vi "Dashboard Main.vi"() -> ()   [LabVIEW 2012]
uses:
  <vilib>/event_ctls.llb/eventvkey.ctl
  <vilib>/Utility/config.llb/Read Key (String).vi
  <vilib>/Utility/config.llb/Read Key (I32).vi
  <vilib>/Utility/config.llb/Write Key (String).vi
  <vilib>/Utility/config.llb/Write Key (I32).vi
  <vilib>/Utility/config.llb/NI_LVConfig.lvlib
panel:
  out "Battery Value":dbl(slide) scale=0.0..14.0 scale format="%#_2e"
  out "Battery":sgl(graph)
  in  "Camera Settings":T1={"Frate Rate"=30, "Compression"=30, "Size"=1} {"Frate Rate" scale=1.0..30.0; "Size" items=["640x480", "320x240", "160x120"]}
  out "Mode":T2(ring)=enum."Auto Disabled"
  out "Camera IP":string
  out "JS1 Z":dbl(slide) scale=-1.0..1.0 scale format="%#_2e"
  out "JS2 Z":dbl(slide) scale=-1.0..1.0 scale format="%#_2e"
  out "Joystick 1":cluster{"X":dbl, "Y":dbl}[](graph)
  out "Joystick 2":cluster{"X":dbl, "Y":dbl}[](graph)
  out "JS Buttons 1":T3
  out "JS Buttons 2":T3
  out "MotorSlide4":dbl(slide) scale=-1.0..1.0 scale format="%#_2e"
  out "MotorSlide3":dbl(slide) scale=-1.0..1.0 scale format="%#_2e"
  out "MotorSlide2":dbl(slide) scale=-1.0..1.0 scale format="%#_2e"
  in  "MotorName3":string="Front Left"
  in  "MotorName4":string="Front Right"
  in  "MotorName1":string="Rear Left"
  in  "MotorName2":string="Rear Right"
  out "MotorChart4":dbl(graph)
  out "MotorChart3":dbl(graph)
  out "MotorChart2":dbl(graph)
  out "MotorSlide1":dbl(slide) scale=-1.0..1.0 scale format="%#_2e"
  out "MotorChart1":dbl(graph)
  out "Robot IP":string
  in  "Dashboard Tab":enum32{"Operation", "Test", "Checklist"}(tab)
  in  "Checkbox 2":bool
  in  "Checkbox 1":bool
  in  "Slider 1":dbl(slide) scale=0.0..100.0
  in  "Slider":dbl(slide) scale=0.0..100.0 scale format="%#_3g"
  in  "On/Off":bool caption="Solenoid"
  in  "Test Name":u16(ring) items=["Select the test to run...", "Example Test", "-------------------------------", "List of tests is built in robot code.", "Replace with your own automated tests."]
  in  "Test Tree":string(tree)
  in  "Motor":cluster{"Value":dbl, "Enable":bool} {"Value" scale=-1.0..1.0 scale format="%#_3g"}
  out "Progress":T4 {"Test Progress" scale=0.0..100.0}
  in  "Rev/Fwd":cluster{"Forward":bool, "Reverse":bool}
  in  "Ring":u16(ring) items=["Auto", "Fixed indoor", "Fixed outdoor 1", "Fixed outdoor 2", "Fixed fluorescent 1", "Fixed fluorescent 2", "Hold current"]
  in  "Listbox":i32(listbox)
  in  "Viewer":T5(tab)
  out "Mbps":dbl format="%#.1g"
  in  "Enable":bool
  in  "DB Camera Config":bool
  out "Mbps":bool
  out "fps":dbl format="%#.1g"
  out "Image Error Message":string="Timeout in Camera Communications"
  out "Camera Image":T6(plugin-control)
  out "Buttons 1":cluster{"1":bool, "2":bool, "3":bool}
  out "Kinect 1":cluster{"X":dbl, "Y":dbl, "Z":dbl} {"X" scale=1.0..-1.0; "Y" scale=1.0..-1.0; "Z" scale=1.0..-1.0}
  out "Buttons 2":cluster{"1":bool, "2":bool, "3":bool}
  out "Kinect 2":cluster{"X":dbl, "Y":dbl, "Z":dbl} {"X" scale=1.0..-1.0; "Y" scale=1.0..-1.0; "Z" scale=1.0..-1.0}
  out "Version":string
  out "Skeleton Picture":picture
  out "Players":i8
  out "Tree":string(tree)
  # "Drive & Motors"
  # "Robot IP:"
  # "Customize by placing controls and indicators here and name to match\nDashboard Variables on robot."
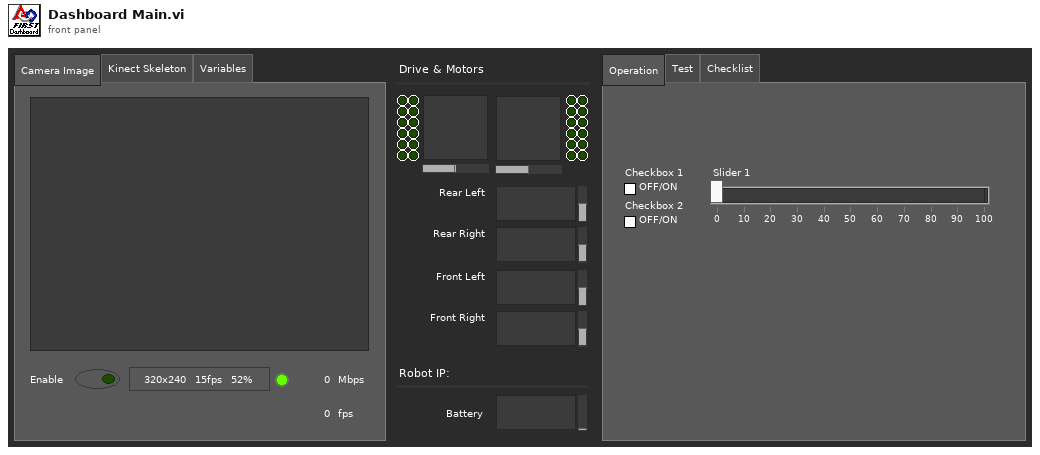
[diagram p1: front panel]
types:
  T1 = cluster{"Frate Rate":i32, "Compression":i32, "Size":u16}
  T2 = enum8{"Tele-Op Disabled", "Tele-Op Enabled", "Auto Disabled", "Auto Enabled", "Test Disabled", "Test Enabled", ""}
  T3 = cluster{bool, bool, bool, bool, bool, bool, bool, bool, bool, bool, bool, bool}
  T4 = cluster{"Test Progress":u8, "Test Progress Text":string}
  T5 = enum32{"Camera Image", "Kinect Skeleton", "Variables"}
  T6 = typedef "IMAQ Image.ctl" = refnum<image>
  T7 = typedef "Image Type" = u32
  T8 = typedef "LVBoundsTypeDef.ctl" = cluster{"Width":u32, "Height":u32}
  T9 = typedef "SkeletonTrackState.ctl" = enum32{"NotTracked", "PositionOnly", "Tracked"}
  T10 = cluster{"TrackingState":u8[], "Position":cluster{"x":sgl, "y":sgl, "z":sgl}, cluster{"x":sgl, "y":sgl, "z":sgl, sgl}[], "TrackState":T9}
  T11 = cluster{cluster{"ScaledToPercentRange":dbl, "ScaledToPercentRange":dbl, "ScaledToPercentRange":dbl}, cluster{bool, bool, bool}}[]
  T12 = cluster{cluster{"ScaledToPercentRange":dbl, "ScaledToPercentRange":dbl, "ScaledToPercentRange":dbl}, cluster{bool, bool, bool}}
  T13 = cluster{"ScaledToPercentRange":dbl, "ScaledToPercentRange":dbl, "ScaledToPercentRange":dbl}
  T14 = typedef "LVRectTypeDef.ctl" = cluster{"Left":i16, "Top":i16, "Right":i16, "Bottom":i16}
  T15 = cluster{"Competition mode":bool, "Robot Link":bool, "Autonomous":bool, "Enabled":bool, "E-Stop":bool, "Simulated":bool, "TestMode":bool, "Docked Window":bool}
  T16 = cluster{"Boolean Array[0]":bool, "Boolean Array[1]":bool, "Boolean Array[2]":bool, "Boolean Array[3]":bool, "Boolean Array[4]":bool, "Boolean Array[5]":bool, "Boolean Array[6]":bool, "Boolean Array[7]":bool, "Boolean Array[8]":bool, "Boolean Array[9]":bool, "Boolean Array[10]":bool, "Boolean Array[11]":bool}
  T17 = typedef "NI_LVConfig.lvlib/Config Data RefNum.ctl" = refnum<k1>
  T18 = typedef "eventvkey.ctl" = enum16{"ASCII", "Enter", "Return", "Shift", "Ctrl", "Alt", "Cmd", "Opt", "Caps", "NumLock", "Clear", "Break", "Up", "Down", "Left", "Right", "Insert", "Delete", "Home", "End", "PageUp", "PageDown", "Escape", "Help", "Pause", "ScrollLock", "F1", "F2", "F3", "F4", "F5", "F6", "F7", "F8", "F9", "F10", "F11", "F12", "F13", "F14", "F15", "F16", "F17", "F18", "F19", "F20", "F21", "F22", "F23", "F24", "Play", "VolumeUp", "VolumeDown", "Mute", "Two Byte Char"}
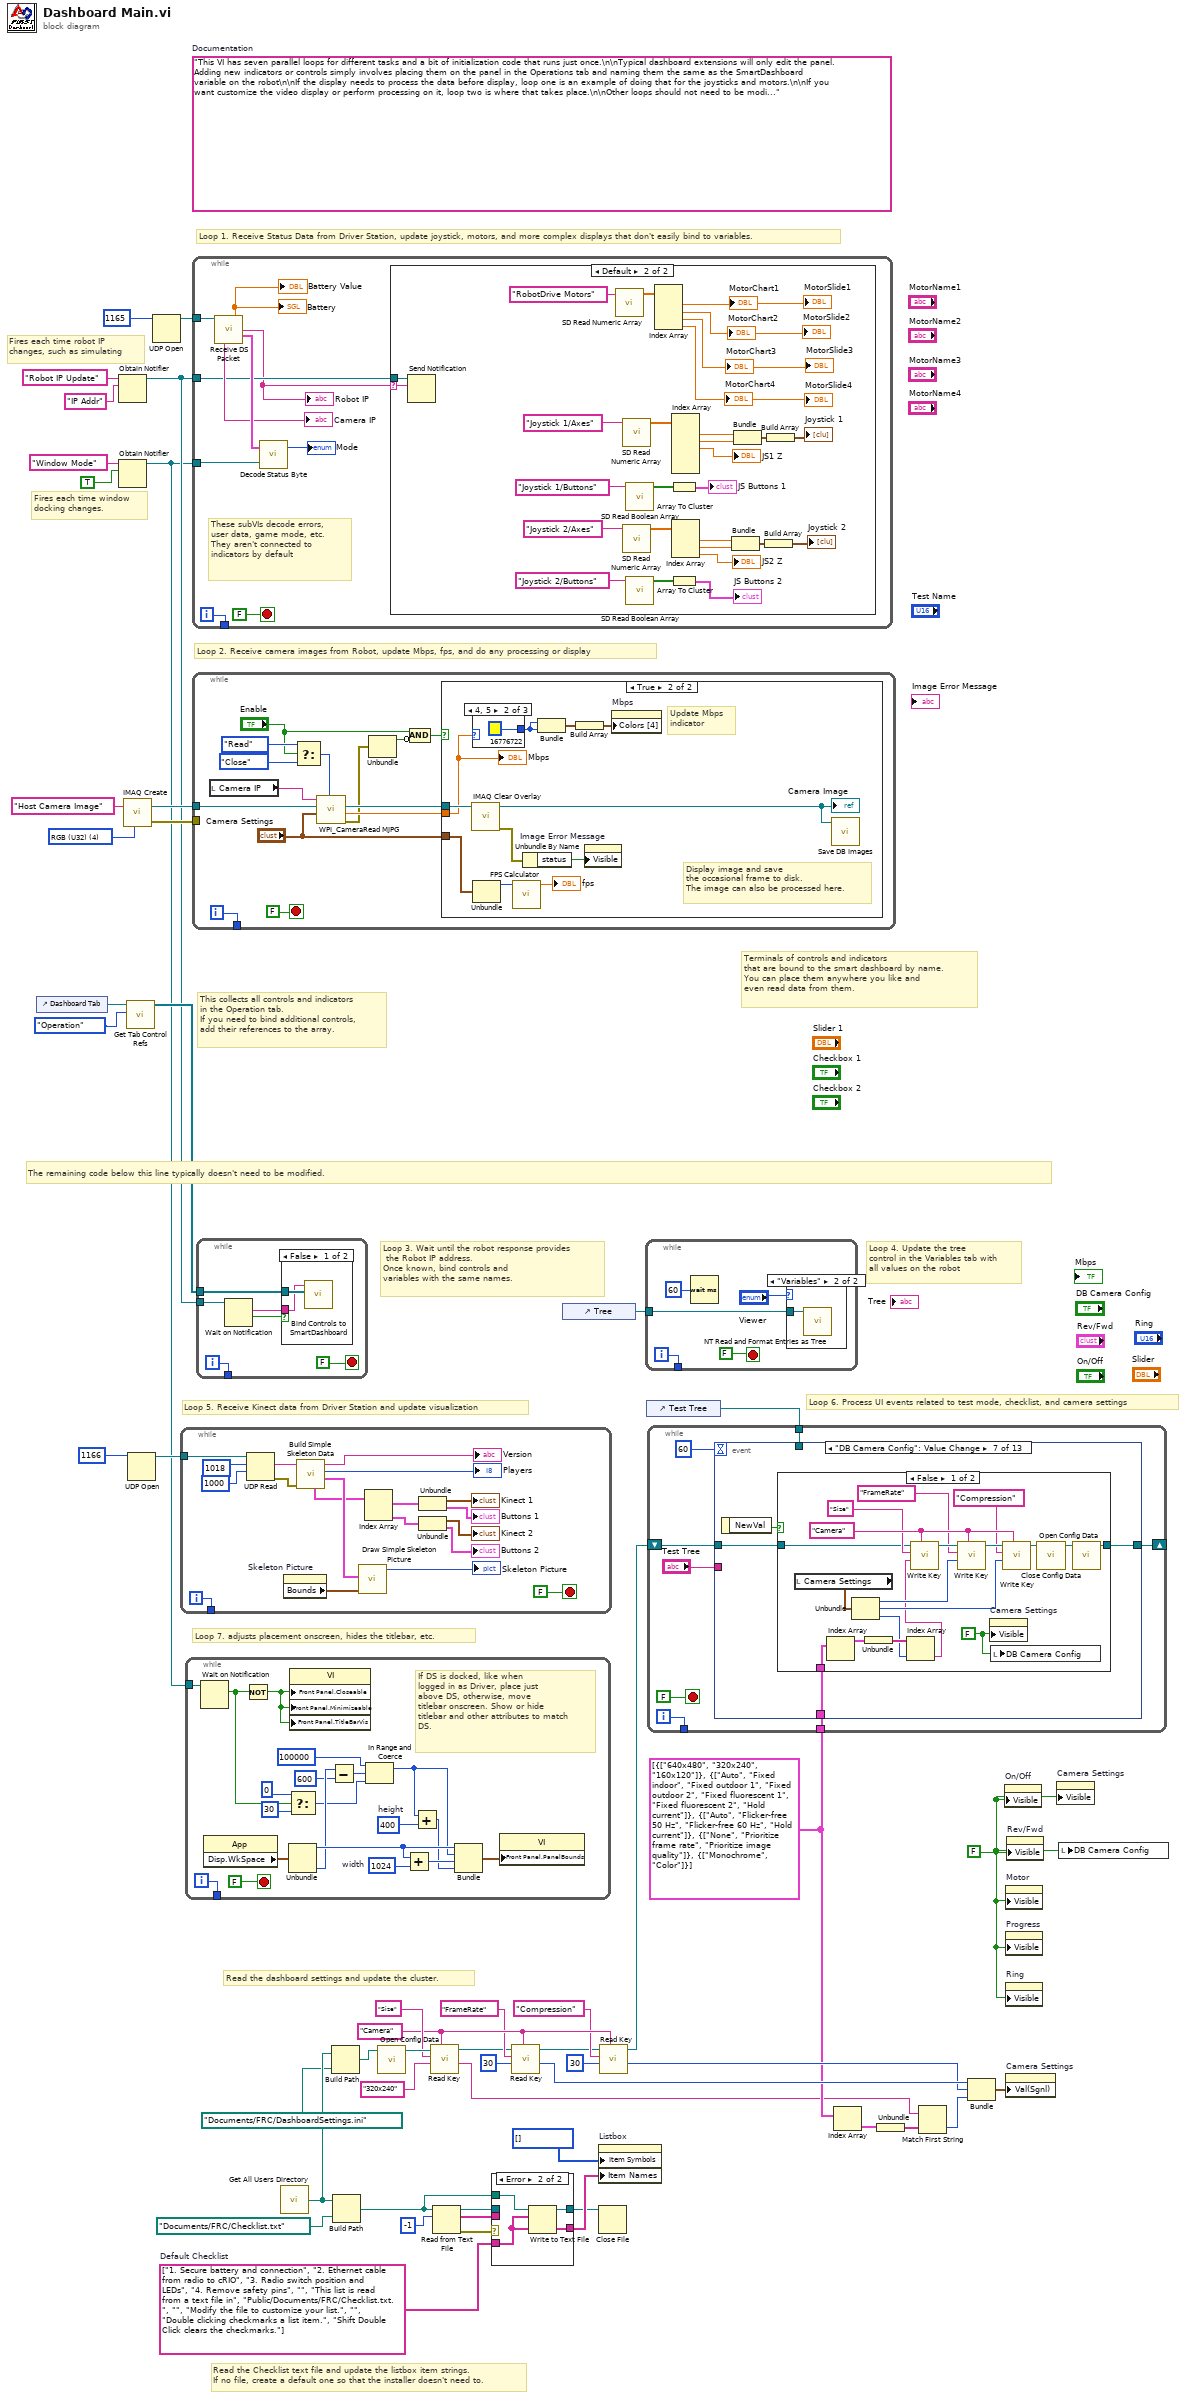
[diagram p0: block diagram]
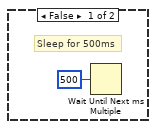
[diagram p3: hidden frame]
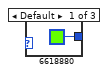
[diagram p4: hidden frame]
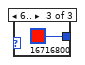
[diagram p5: hidden frame]
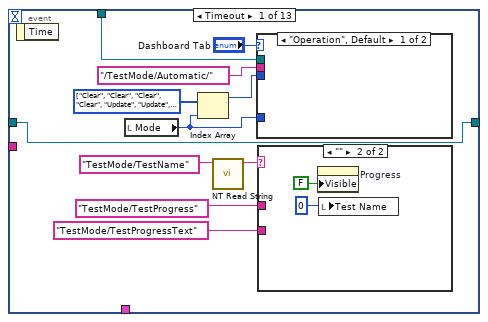
[diagram p7: hidden frame]
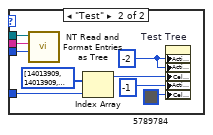
[diagram p8: hidden frame]
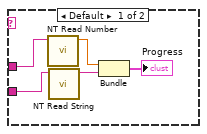
[diagram p9: hidden frame]
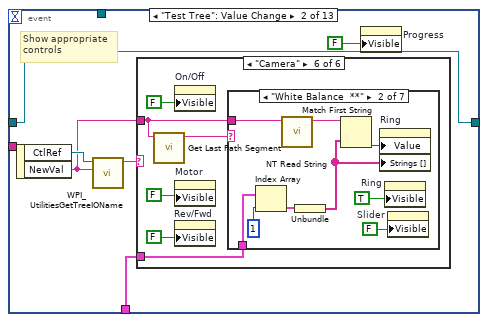
[diagram p10: hidden frame]
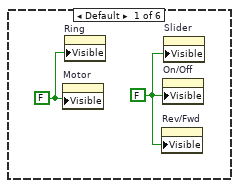
[diagram p11: hidden frame]
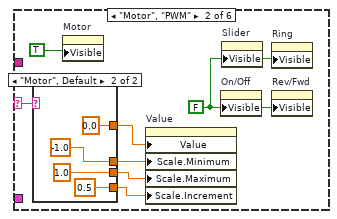
[diagram p12: hidden frame]
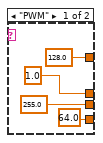
[diagram p13: hidden frame]
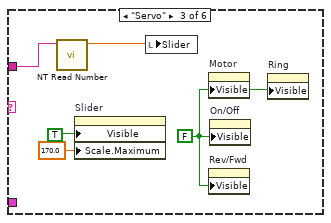
[diagram p14: hidden frame]
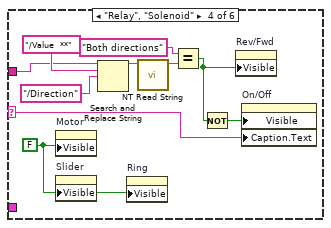
[diagram p15: hidden frame]
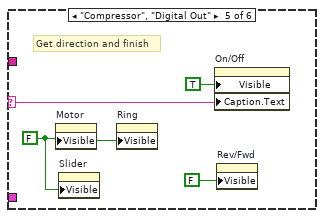
[diagram p16: hidden frame]
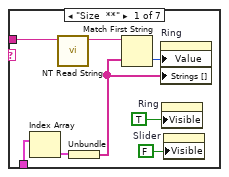
[diagram p17: hidden frame]
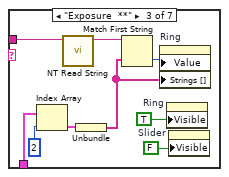
[diagram p18: hidden frame]
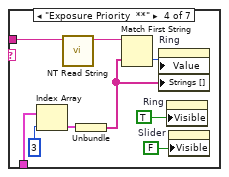
[diagram p19: hidden frame]
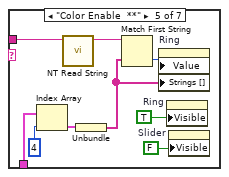
[diagram p20: hidden frame]
diagram:
  w21 = "Camera"
  w13 = cluster{string[]}[] [{["640x480", "320x240", "160x120"]}, {["Auto", "Fixed indoor", "Fixed outdoor 1", "Fixed outdoor 2", "Fixed fluorescent 1", "Fixed fluorescent 2", "Hold current"]}, {["Auto", "Flicker-free 50 Hz", "Flicker-free 60 Hz", "Hold current"]}, {["None", "Prioritize frame rate", "Prioritize image quality"]}, {["Monochrome", "Color"]}]
  w29 = string[] ["1. Secure battery and connection", "2. Ethernet cable from radio to cRIO", "3. Radio switch position and LEDs", "4. Remove safety pins", "", "This list is read from a text file in", "Public/Documents/FRC/Checklist.txt.", "", "Modify the file to customize your list.", "", "Double clicking checkmarks a list item.", "Shift Double Click clears the checkmarks."]  # Default Checklist
  w27 = FALSE ("Visible")
  (unwired) "This VI has seven parallel loops for different tasks and a bit of initialization code that runs just once.\n\nTypical dashboard extensions will only edit the panel. Adding new indicators or controls simply involves placing them on the panel in the Operations tab and naming them the same as the SmartDashboard variable on the robot\n\nIf the display needs to process the data before display, loop one is an example of doing that for the joysticks and motors.\n\nIf you want customize the video display or perform processing on it, loop two is where that takes place.\n\nOther loops should not need to be modified. They are pretty standard, and document the task they perform."  # Documentation
  w50 = T7 4 items=["Grayscale (U8)", "Grayscale (I16)", "Grayscale (SGL)", "Complex (CSG)", "RGB (U32)", "HSL (U32)", "RGB (U64)"] ("Image Type")
  # "Fires each time robot IP\nchanges, such as simulating"
  # "Fires each time window\ndocking changes."
  # "Read the Checklist text file and update the listbox item strings.\nIf no file, create a default one so that the installer doesn't need to."
  # "This collects all controls and indicators\nin the Operation tab.\nIf you need to bind additional controls,\nadd their references to the array."
  # "The remaining code below this line typically doesn't need to be modified."
  # "Loop 6. Process UI events related to test mode, checklist, and camera settings"
  # "Read the dashboard settings and update the cluster."
  # "Terminals of controls and indicators\nthat are bound to the smart dashboard by name.\nYou can place them anywhere you like and\neven read data from them."
  # "Loop 4. Update the tree\ncontrol in the Variables tab with\nall values on the robot"
  # "Loop 3. Wait until the robot response provides\n the Robot IP address.\nOnce known, bind controls and\nvariables with the same names."
  # "Loop 5. Receive Kinect data from Driver Station and update visualization"
  # "Loop 7. adjusts placement onscreen, hides the titlebar, etc."
  # "Loop 1. Receive Status Data from Driver Station, update joystick, motors, and more complex displays that don't easily bind to variables."
  # "Loop 2. Receive camera images from Robot, update Mbps, fps, and do any processing or display"
  n1 = control-ref of="Dashboard Tab"() -> (w43:refnum<vi>)
  n2 = Obtain Notifier(name (unnamed)="Robot IP Update", notification data type="IP Addr" ("name (unnamed)")) -> (notifier out=w40:refnum<notifier>)  [unwired: 2 in, 2 out]
  n3 = Obtain Notifier(name (unnamed)="Window Mode", notification data type=TRUE) -> (notifier out=w33:refnum<notifier>)  [unwired: 2 in, 2 out]
  n4 = call "IMAQ Create"("Image Name"="Host Camera Image", "Image Type"=w50) -> ("New Image"=w48:T6, "error out"=w47:errorcluster)  [unwired: 2 in, 1 out]
  n5 = call <vilib>:"Get Tab Control Refs.vi"("Page Index"=enum32{"Operation", "Test"}."Operation" ("Dashboard Tab"), "TabControl in"=w43) -> ("ControlsOnPage"=w44:refnum<vi>[])  [unwired: 9 in]
  n6 = UDP Open(11:u16 1166 ("port")) -> (port=w45:refnum<k16>)  [unwired: 2 in, 4 out]
  n7 = UDP Open(11:u16 1165 ("port")) -> (port=w51:refnum<k16>)  [unwired: 2 in, 4 out]
  n8 = while {
    tunnel: w45 -> [w69]
    tunnel: [w54] -> _
    i -> [w54]
    stop <- FALSE stop-if-true
    n9 = UDP Read(connection ID=w69, max size (548)=1018 ("bytes to read"), timeout ms (25000)=1000) -> (data out=w63:string, error out=w53:errorcluster)  [unwired: 1 in, 3 out]
    n10 = property on="Skeleton Picture" class="Pict"() -> ("Bounds"=w65:T8)  [unwired: 2 in, 2 out]
    n11 = call "Build Simple Skeleton Data.vi"("error in (no error)"=w53, "data in"=w63) -> ("Skeleton Data"=w64:T10, "NumPlayers"=→"Players":i8, "Version String"=→"Version":string, "Simple Joystick Info"=w61:T11)  [unwired: 5 in, 1 out]
    n12 = call "Draw Simple Skeleton Picture.vi"("Bounds"=w65, "Simple Skeleton"=w64) -> ("new picture out"=→"Skeleton Picture":picture)  [unwired: 9 in]
    n13 = Index Array(array=w61) -> (element #1=w60:T12, element #2=w59:T12)  [unwired: 2 in]
    n14 = Unbundle(w60) -> (→"Kinect 1":T13, →"Buttons 1":cluster{bool, bool, bool})
    n15 = Unbundle(w59) -> (→"Kinect 2":T13, →"Buttons 2":cluster{bool, bool, bool})
  }
  n16 = while {
    tunnel: w33 -> [w90]
    tunnel: [w88] -> _
    i -> [w88]
    stop <- FALSE stop-if-true
    w80 = 1024  # width
    w83 = 400  # height
    # "If DS is docked, like when\nlogged in as Driver, place just\nabove DS, otherwise, move\ntitlebar onscreen. Show or hide\ntitlebar and other attributes to match\nDS."
    n17 = Wait on Notification(notifier=w90) -> (notification=w75:bool)  [unwired: 3 in, 3 out]
    n18 = property class="App"() -> ("Disp.WkSpace"=w86:T14)  [unwired: 2 in, 2 out]
    n19 = Not(x=w75) -> (.not. x?=w89:bool)
    n20 = Unbundle(w86) -> ("Left"=w84:i16, "Bottom"=w81:i16)  [unwired: 2 out]
    n21 = Select(t=0, s=w75, f=30) -> (s? t:f=w74:i32)
    n22 = property class="VI"("Front Panel.Closeable"=w89, "Front Panel.Minimizeable"=w89, "Front Panel.TitleBarVis"=w89) -> ()  [unwired: 2 in, 2 out]
    n23 = Subtract(x=w81, y=600) -> (x-y=w78:i32)
    n24 = In Range and Coerce(upper limit=100000, x=w78, lower limit=w74) -> (coerced(x)=w72:i32)  [unwired: 1 out]
    n25 = Add(x=w84, y=w80) -> (x+y=w85:i32)
    n26 = Add(x=w72, y=w83) -> (x+y=w82:i32)
    n27 = Bundle("Left"=w84, w72, w85, w82) -> (w87:cluster{"Left":i16, i32, i32, i32})  [unwired: 1 out]
    n28 = property class="VI"("Front Panel.PanelBounds"=w87) -> ()  [unwired: 2 in, 2 out]
  }
  n29 = while {
    tunnel: w48 -> [w101]
    tunnel: w47 -> [_]
    tunnel: [w104] -> _
    i -> [w104]
    stop <- FALSE stop-if-true
    n30 = local read "Camera IP"() -> (w103:string)
    n31 = Select(t=enum16{"Read", "Reopen", "Close"}."Read" ("Operation"), s="Enable", f=enum16{"Read", "Reopen", "Close"}."Close" ("Operation")) -> (s? t:f=w96:enum16{"Read", "Reopen", "Close"})
    n32 = call <vilib>:"WPI_CameraRead MJPG.vi"("Operation"=w96, "Camera Settings"="Camera Settings", "Image"=w101, "address"=w103) -> ("error out"=w95:errorcluster, "Bandwidth (kbps)"=w99:dbl, "Image Out"=w100:T6)  [unwired: 5 in]
    n33 = Unbundle(w95) -> ("status"=w93:bool)  [unwired: 2 out]
    n34 = Compound Arithmetic op=AND("Enable", invert w93) -> (w92:bool)
    n35 = case shown="True" w92 {
      tunnel: "Camera Settings" -> [_ w108]
      tunnel: w100 -> [_ w111]
      tunnel: w99 -> [_ w110]
      frame False {
        # "Sleep for 500ms"
        n36 = Wait Until Next ms Multiple(millisecond multiple=u32 500) -> ()  [unwired: 1 out]
      }
      frame True {
        # "Display image and save\nthe occasional frame to disk.\nThe image can also be processed here."
        # "Update Mbps\nindicator"
        n37 = call "IMAQ Clear Overlay"("Image"=w111) -> ("error out"=w116:errorcluster, "Image Out"=w115:T6)  [unwired: 2 in, 7 out]
        "Camera Image" <- w115
        n38 = case shown="4, 5" w110 {
          tunnel: [u32 6618880 ("Color Box") u32 16776722 ("Color Box") u32 16716800 ("Color Box")] -> w112
          frame Default {
          }
          frame 4, 5 {
          }
          frame 6.. {
          }
        }
        n39 = Unbundle(w108) -> ("Frate Rate"=w107:i32)  [unwired: 2 out]
        n40 = call "FPS Calculator.vi"("Average Count"=w107) -> ("fps"=→"fps":dbl)  [unwired: 10 in]
        n41 = Unbundle By Name(w116) -> ("status"=w117:bool)
        n42 = Bundle("Color Box"=w112, "Color Box"=w112) -> (w114:cluster{"Color Box":u32, "Color Box":u32})  [unwired: 1 out]
        n43 = Build Array(w114) -> (w113:cluster{"Color Box":u32, "Color Box":u32}[])
        n44 = property on="Image Error Message" class="Str"("Visible"=w117) -> ()  [unwired: 2 in, 2 out]
        n45 = property on="Mbps" class="Bool (strict)"("Colors [4]"=w113) -> ()  [unwired: 2 in, 2 out]
        n46 = call "Save DB Images.vi"("Image"=w115) -> ()  [unwired: 2 in, 1 out]
        "Mbps" <- w110
      }
    }
  }
  n47 = while {
    tunnel: w51 -> [w128]
    tunnel: w40 -> [w122]
    tunnel: w33 -> [w126]
    tunnel: [w123] -> _
    i -> [w123]
    stop <- FALSE stop-if-true
    # "These subVIs decode errors, user data, game mode, etc.\nThey aren't connected to indicators by default"
    n48 = call "Receive DS Packet.vi"("Recv Socket"=w128) -> ("Battery"=→"Battery" →"Battery Value":sgl, "Robot IP Address"=w121:string, "Status"=w129:T15, "Camera IP Address"=→"Camera IP":string)  [unwired: 1 in, 10 out]
    "Robot IP" <- w121
    n49 = call "Decode Status Byte.vi"("Window Mode Notifier"=w126, "Status"=w129) -> ("Mode"=→"Mode":T2)  [unwired: 1 out]
    n50 = case shown="Default" w121 {
      selector: w121 -> [_ w131]
      tunnel: w122 -> [_ w132]
      frame "0.0.0.0" {
        # "Robot not responding, don't poll the variables"
      }
      frame Default {
        n51 = Send Notification(notification=w131, notifier=w132) -> ()  [unwired: 1 in, 2 out]
        n52 = call <vilib>:"SD Read Numeric Array.vi"("Name"="RobotDrive Motors") -> ("Numeric Array"=w155:dbl[])  [unwired: 8 in, 2 out]
        n53 = call <vilib>:"SD Read Numeric Array.vi"("Name"="Joystick 1/Axes") -> ("Numeric Array"=w148:dbl[])  [unwired: 8 in, 2 out]
        n54 = call <vilib>:"SD Read Numeric Array.vi"("Name"="Joystick 2/Axes") -> ("Numeric Array"=w142:dbl[])  [unwired: 8 in, 2 out]
        n55 = call <vilib>:"SD Read Boolean Array.vi"("Name"="Joystick 1/Buttons") -> ("Boolean Array"=w150:bool[])  [unwired: 8 in, 2 out]
        n56 = call <vilib>:"SD Read Boolean Array.vi"("Name"="Joystick 2/Buttons") -> ("Boolean Array"=w141:bool[])  [unwired: 8 in, 2 out]
        n57 = Index Array(array=w155) -> (element #1=→"MotorChart1" →"MotorSlide1":dbl, element #2=→"MotorSlide2" →"MotorChart2":dbl, element #3=→"MotorChart3" →"MotorSlide3":dbl, element #4=→"MotorChart4" →"MotorSlide4":dbl)  [unwired: 4 in]
        n58 = Array To Cluster(array=w150) -> (cluster=→"JS Buttons 1":T16)
        n59 = Array To Cluster(array=w141) -> (cluster=→"JS Buttons 2":T16)
        n60 = Index Array(array=w148) -> (element #1=w145:dbl, element #2=w146:dbl, element #3=→"JS1 Z":dbl)  [unwired: 6 in, 3 out]
        n61 = Index Array(array=w142) -> (element #1=w137:dbl, element #2=w136:dbl, element #3=→"JS2 Z":dbl)  [unwired: 3 in]
        n62 = Bundle("Numeric"=w137, "Numeric"=w136) -> (w138:cluster{"Numeric":dbl, "Numeric":dbl})  [unwired: 1 in]
        n63 = Bundle("Numeric"=w145, "Numeric"=w146) -> (w144:cluster{"Numeric":dbl, "Numeric":dbl})  [unwired: 1 in]
        n64 = Build Array(w138) -> (→"Joystick 2":cluster{"Numeric":dbl, "Numeric":dbl}[])
        n65 = Build Array(w144) -> (→"Joystick 1":cluster{"Numeric":dbl, "Numeric":dbl}[])
      }
    }
  }
  n66 = while {
    tunnel: w44 -> [w164]
    tunnel: w40 -> [w161]
    tunnel: [w159] -> _
    i -> [w159]
    stop <- FALSE stop-if-true
    n67 = Wait on Notification(notifier=w161) -> (notification=w160:string, timed out?=w162:bool)  [unwired: 3 in, 2 out]
    n68 = case shown="False" w162 {
      tunnel: w164 -> [w166 _]
      tunnel: w160 -> [w165 _]
      frame False {
        n69 = call <vilib>:"Bind Controls to SmartDashboard.vi"("Bound Control Refs"=w166, "Server IP Address"=w165) -> ()  [unwired: 10 in]
      }
      frame True {
      }
    }
  }
  n70 = call "Get All Users Directory.vi"() -> ("All User Path"=w26:path)
  n71 = Build Path(base path=w26, name or relative path=path "Documents/FRC/DashboardSettings.ini") -> (appended path=w25:path)
  n72 = Build Path(base path=w26, name or relative path=path "Documents/FRC/Checklist.txt") -> (appended path=w30:path)
  n73 = call <vilib>:"Open Config Data.vi"("configuration file path"=w25) -> ("refnum"=w24:T17)  [unwired: 8 in, 2 out]
  n74 = call-poly <vilib>:"Read Key.vi"("section"=w21, "default value"="320x240", "key"="Size", "refnum"=w24) -> ("value"=w11:string, "refnum out"=w6:T17)  [unwired: 2 in, 4 out]
  n75 = Read from Text File(file (use dialog)=w30, count=-1 ("timeout ms (25000)")) -> (refnum out=w8:refnum<file>, text=w31:string[], error out=w32:errorcluster)  [unwired: 2 in, 1 out]
  n76 = case shown="Error" w32 {
    tunnel: w31 -> [w168 _]
    tunnel: [w168 w170] -> w28
    tunnel: w29 -> [_ w170]
    tunnel: w30 -> [_ w171]
    tunnel: [w167 w169] -> w7
    tunnel: w8 -> [w167 _]
    frame No Error {
    }
    frame Error {
      n77 = Write to Text File(file (use dialog)=w171, text=w170) -> (refnum out=w169:refnum<file>)  [unwired: 2 in, 2 out]
    }
  }
  n78 = call-poly <vilib>:"Read Key.vi"("section"=w21, "default value"=30, "key"="FrameRate", "refnum"=w6) -> ("value"=w16:i32, "refnum out"=w5:T17)  [unwired: 1 in, 5 out]
  n79 = control-ref of="Tree"() -> (w2:refnum<vi>)
  n80 = property on="Listbox" class="LstBox (strict)"("Item Symbols"=i32[] [], "Item Names"=w28) -> ()  [unwired: 2 in, 2 out]
  n81 = Close File(refnum=w7) -> ()  [unwired: 1 in, 2 out]
  n82 = call-poly <vilib>:"Read Key.vi"("section"=w21, "default value"=30, "key"="Compression", "refnum"=w5) -> ("value"=w15:i32, "refnum out"=w3:T17)  [unwired: 1 in, 5 out]
  n83 = while {
    tunnel: [w173] -> _
    tunnel: w2 -> [w172]
    i -> [w173]
    stop <- FALSE stop-if-true
    n84 = Wait (ms)(milliseconds to wait=u32 60) -> ()  [unwired: 1 out]
    n85 = case shown="\"Variables\"" "Viewer" {
      tunnel: w172 -> [_ w177]
      frame Default {
      }
      frame "Variables" {
        n86 = call <vilib>:"NT Read and Format Entries as Tree.vi"("Tree Refnum"=w177) -> ()  [unwired: 9 in, 2 out]
      }
    }
  }
  n87 = control-ref of="Test Tree"() -> (w1:refnum<vi>)
  n88 = while {
    tunnel: w13 -> [w182]
    shift-right: [w181] -> _
    shift-left: w3 -> [w180]
    tunnel: [w179] -> _
    tunnel: w1 -> [w178]
    i -> [w179]
    stop <- FALSE stop-if-true
    n89 = event shown="[6] \"DB Camera Config\": Value Change" {
      selector: _ -> [_ _ _ _ _ _ _ _ _ _ _ _ _]
      dyn-events: _ -> [_ _ _ _ _ _ _ _ _ _ _ _ _]
      timeout: u32 60 ("milliseconds to wait") -> [_ _ _ _ _ _ _ _ _ _ _ _ _]
      tunnel: w178 -> [w192 _ _ _ _ _ _ _ _ _ _ _ _]
      tunnel: "Test Tree" -> [_ _ _ _ _ _ _ _ w386 w394 w396 w400 w408]
      tunnel: w182 -> [_ w214 _ _ _ _ w350 w380 _ _ _ _ _]
      tunnel: [w186 w213 _ w316 w324 w336 w349 w373 w385 w392 w395 w399 w407] -> w181
      tunnel: w180 -> [w186 w213 _ w316 w324 w336 w348 w373 w385 w392 w395 w399 w407]
      event Timeout {
        w191 = enum16{"Update", "Clear"}[] [enum."Clear", enum."Clear", enum."Clear", enum."Clear", enum."Update", enum."Update", enum."Clear"] items=["Update", "Clear"]
        n90 = event-data() -> ()  [unwired: 1 in, 1 out]
        n91 = local read "Mode"() -> (w189:T2)
        n92 = Index Array(array=w191, index=w189) -> (element=w190:enum16{"Update", "Clear"})
        n93 = call <vilib>:"NT Read String.vi"("Name"="TestMode/TestName") -> ("String"=w195:string)  [unwired: 9 in, 1 out]
        n94 = case shown="\"Operation\", Default" "Dashboard Tab" {
          tunnel: w192 -> [_ w205]
          tunnel: "/TestMode/Automatic/" ("Name Pattern") -> [_ w204]
          tunnel: w190 -> [_ w203]
          tunnel: w189 -> [_ w201]
          frame "Operation", Default {
          }
          frame "Test" {
            w200 = -2 ("Active Item:Row Number")
            n95 = call <vilib>:"NT Read and Format Entries as Tree.vi"("Operation"=w203, "Name Pattern"=w204, "Tree Refnum"=w205) -> ()  [unwired: 7 in, 2 out]
            n96 = Index Array(array=u32[] [14013909, 14013909, 14013909, 14013909, 14013909, 16777215, 14013909], index=w201) -> (element=w199:u32)
            n97 = property on="Test Tree" class="Tree (strict)"("Active Item Row Number"=w200, "ActiveColNum"=w200, "CellBG"=w199, "Active Item Row Number"=-1 ("Active Item:Row Number"), "CellBG"=u32 5789784 ("Color Box")) -> ()  [unwired: 2 in, 2 out]
          }
        }
        n98 = case shown="\"\"" w195 {
          tunnel: "TestMode/TestProgress" ("Name") -> [w207 _]
          tunnel: "TestMode/TestProgressText" ("Name") -> [w206 _]
          frame Default {
            n99 = call <vilib>:"NT Read Number.vi"("Name"=w207) -> ("Numeric"=w208:dbl)  [unwired: 9 in, 1 out]
            n100 = call <vilib>:"NT Read String.vi"("Name"=w206) -> ("String"=w209:string)  [unwired: 9 in, 1 out]
            n101 = Bundle("Numeric"=w208, "String"=w209) -> (→"Progress":cluster{"Numeric":dbl, "String":string})  [unwired: 1 in]
          }
          frame "" {
            n102 = property on="Progress" class="Clust (strict)"("Visible"=FALSE) -> ()  [unwired: 2 in, 2 out]
            n103 = local write "Test Name"(u16 0) -> ()
          }
        }
      }
      event "Test Tree": Value Change {
        # "Show appropriate\ncontrols"
        n104 = event-data() -> ("CtlRef"=w217:refnum<vi>, "NewVal"=w215:string)  [unwired: 1 in]
        n105 = call <vilib>:"WPI_UtilitiesGetTreeIOName.vi"("NewVal"=w215, "TreeControl in"=w217) -> ("I/O Name"=w218:string)  [unwired: 9 in]
        n106 = case shown="\"Camera\"" w218 {
          selector: w218 -> [_ w225 _ w243 w252 _]
          tunnel: w215 -> [_ _ w240 w242 _ w259]
          tunnel: w214 -> [_ _ _ _ _ w258]
          frame Default {
            w220 = FALSE ("Visible")
            w219 = FALSE ("Visible")
            n107 = property on="Motor" class="Clust (strict)"("Visible"=w219) -> ()  [unwired: 2 in, 2 out]
            n108 = property on="Ring" class="Ring (strict)"("Visible"=w219) -> ()  [unwired: 2 in, 2 out]
            n109 = property on="Rev/Fwd" class="Clust (strict)"("Visible"=w220) -> ()  [unwired: 2 in, 2 out]
            n110 = property on="On/Off" class="Bool (strict)"("Visible"=w220) -> ()  [unwired: 2 in, 2 out]
            n111 = property on="Slider" class="Slide (strict)"("Visible"=w220) -> ()  [unwired: 2 in, 2 out]
          }
          frame "Motor", "PWM" {
            w226 = FALSE ("Visible")
            n112 = case shown="\"Motor\", Default" w225 {
              tunnel: [1.0 ("Value") -1.0 ("Value")] -> w224
              tunnel: [255.0 ("Value") 1.0 ("Value")] -> w223
              tunnel: [128.0 ("Value") 0.0 ("Value")] -> w222
              tunnel: [64.0 ("Value") 0.5 ("Value")] -> w221
              frame "PWM" {
              }
              frame "Motor", Default {
              }
            }
            n113 = property on="Motor" class="Clust (strict)"("Visible"=TRUE) -> ()  [unwired: 2 in, 2 out]
            n114 = property on="Value" class="Slide (strict)"("Value"=w222, "Scale.Minimum"=w224, "Scale.Maximum"=w223, "Scale.Increment"=w221) -> ()  [unwired: 2 in, 2 out]
            n115 = property on="On/Off" class="Bool (strict)"("Visible"=w226) -> ()  [unwired: 2 in, 2 out]
            n116 = property on="Slider" class="Slide (strict)"("Visible"=w226) -> ()  [unwired: 2 in, 2 out]
            n117 = property on="Ring" class="Ring (strict)"("Visible"=w226) -> ()  [unwired: 2 in, 2 out]
            n118 = property on="Rev/Fwd" class="Clust (strict)"("Visible"=w226) -> ()  [unwired: 2 in, 2 out]
          }
          frame "Servo" {
            w238 = FALSE ("Visible")
            n119 = call <vilib>:"NT Read Number.vi"("Name"=w240) -> ("Numeric"=w239:dbl)  [unwired: 9 in, 1 out]
            n120 = property on="Slider" class="Slide (strict)"("Visible"=TRUE, "Scale.Maximum"=170.0 ("Scale.Range:Maximum")) -> ()  [unwired: 2 in, 2 out]
            n121 = local write "Slider"(w239) -> ()
            n122 = property on="Motor" class="Clust (strict)"("Visible"=w238) -> ()  [unwired: 2 in, 2 out]
            n123 = property on="Rev/Fwd" class="Clust (strict)"("Visible"=w238) -> ()  [unwired: 2 in, 2 out]
            n124 = property on="On/Off" class="Bool (strict)"("Visible"=w238) -> ()  [unwired: 2 in, 2 out]
            n125 = property on="Ring" class="Ring (strict)"("Visible"=w238) -> ()  [unwired: 2 in, 2 out]
          }
          frame "Relay", "Solenoid" {
            w241 = FALSE ("Visible")
            n126 = property on="Motor" class="Clust (strict)"("Visible"=w241) -> ()  [unwired: 2 in, 2 out]
            n127 = property on="Slider" class="Slide (strict)"("Visible"=w241) -> ()  [unwired: 2 in, 2 out]
            n128 = Search and Replace String(input string=w242, search string="/Value  **", replace string="/Direction") -> (result string=w248:string)  [unwired: 5 in, 3 out]
            n129 = property on="Ring" class="Ring (strict)"("Visible"=w241) -> ()  [unwired: 2 in, 2 out]
            n130 = call <vilib>:"NT Read String.vi"("Name"=w248) -> ("String"=w246:string)  [unwired: 9 in, 1 out]
            n131 = Equal?(x="Both directions", y=w246) -> (x = y?=w244:bool)
            n132 = Not(x=w244) -> (.not. x?=w245:bool)
            n133 = property on="Rev/Fwd" class="Clust (strict)"("Visible"=w244) -> ()  [unwired: 2 in, 2 out]
            n134 = property on="On/Off" class="Bool (strict)"("Visible"=w245, "Caption.Text"=w243) -> ()  [unwired: 2 in, 2 out]
          }
          frame "Compressor", "Digital Out" {
            w251 = FALSE ("Visible")
            # "Get direction and finish"
            n135 = property on="Motor" class="Clust (strict)"("Visible"=w251) -> ()  [unwired: 2 in, 2 out]
            n136 = property on="Slider" class="Slide (strict)"("Visible"=w251) -> ()  [unwired: 2 in, 2 out]
            n137 = property on="Ring" class="Ring (strict)"("Visible"=w251) -> ()  [unwired: 2 in, 2 out]
            n138 = property on="On/Off" class="Bool (strict)"("Visible"=TRUE, "Caption.Text"=w252) -> ()  [unwired: 2 in, 2 out]
            n139 = property on="Rev/Fwd" class="Clust (strict)"("Visible"=FALSE) -> ()  [unwired: 2 in, 2 out]
          }
          frame "Camera" {
            n140 = call <vilib>:"Get Last Path Segment.vi"("String in"=w259) -> ("String out"=w260:string)  [unwired: 10 in]
            n141 = property on="On/Off" class="Bool (strict)"("Visible"=FALSE) -> ()  [unwired: 2 in, 2 out]
            n142 = property on="Motor" class="Clust (strict)"("Visible"=FALSE) -> ()  [unwired: 2 in, 2 out]
            n143 = property on="Rev/Fwd" class="Clust (strict)"("Visible"=FALSE) -> ()  [unwired: 2 in, 2 out]
            n144 = case shown="\"White Balance  **\"" w260 {
              tunnel: w259 -> [w266 w275 w284 w293 w302 _ w308]
              tunnel: w258 -> [w264 w272 w281 w290 w299 _ _]
              frame "Size  **" {
                n145 = Index Array(array=w264) -> (element=w263:cluster{string[]})  [unwired: 1 in]
                n146 = call <vilib>:"NT Read String.vi"("Name"=w266) -> ("String"=w265:string)  [unwired: 9 in, 1 out]
                n147 = Unbundle(w263) -> (w261:string[])
                n148 = Match First String(2:w261, 3:w265) -> (0:w262:i32)  [unwired: 1 out]
                n149 = property on="Ring" class="Ring (strict)"("Value"=w262, "Strings []"=w261) -> ()  [unwired: 2 in, 2 out]
                n150 = property on="Ring" class="Ring (strict)"("Visible"=TRUE) -> ()  [unwired: 2 in, 2 out]
                n151 = property on="Slider" class="Slide (strict)"("Visible"=FALSE) -> ()  [unwired: 2 in, 2 out]
              }
              frame "White Balance  **" {
                n152 = Index Array(array=w272, index=1) -> (element=w273:cluster{string[]})
                n153 = call <vilib>:"NT Read String.vi"("Name"=w275) -> ("String"=w274:string)  [unwired: 9 in, 1 out]
                n154 = Unbundle(w273) -> (w270:string[])
                n155 = Match First String(2:w270, 3:w274) -> (0:w269:i32)  [unwired: 1 out]
                n156 = property on="Ring" class="Ring (strict)"("Value"=w269, "Strings []"=w270) -> ()  [unwired: 2 in, 2 out]
                n157 = property on="Ring" class="Ring (strict)"("Visible"=TRUE) -> ()  [unwired: 2 in, 2 out]
                n158 = property on="Slider" class="Slide (strict)"("Visible"=FALSE) -> ()  [unwired: 2 in, 2 out]
              }
              frame "Exposure  **" {
                n159 = Index Array(array=w281, index=2) -> (element=w282:cluster{string[]})
                n160 = call <vilib>:"NT Read String.vi"("Name"=w284) -> ("String"=w283:string)  [unwired: 9 in, 1 out]
                n161 = Unbundle(w282) -> (w278:string[])
                n162 = Match First String(2:w278, 3:w283) -> (0:w279:i32)  [unwired: 1 out]
                n163 = property on="Ring" class="Ring (strict)"("Value"=w279, "Strings []"=w278) -> ()  [unwired: 2 in, 2 out]
                n164 = property on="Ring" class="Ring (strict)"("Visible"=TRUE) -> ()  [unwired: 2 in, 2 out]
                n165 = property on="Slider" class="Slide (strict)"("Visible"=FALSE) -> ()  [unwired: 2 in, 2 out]
              }
              frame "Exposure Priority  **" {
                n166 = Index Array(array=w290, index=3) -> (element=w291:cluster{string[]})
                n167 = call <vilib>:"NT Read String.vi"("Name"=w293) -> ("String"=w292:string)  [unwired: 9 in, 1 out]
                n168 = Unbundle(w291) -> (w287:string[])
                n169 = Match First String(2:w287, 3:w292) -> (0:w288:i32)  [unwired: 1 out]
                n170 = property on="Ring" class="Ring (strict)"("Value"=w288, "Strings []"=w287) -> ()  [unwired: 2 in, 2 out]
                n171 = property on="Ring" class="Ring (strict)"("Visible"=TRUE) -> ()  [unwired: 2 in, 2 out]
                n172 = property on="Slider" class="Slide (strict)"("Visible"=FALSE) -> ()  [unwired: 2 in, 2 out]
              }
              frame "Color Enable  **" {
                n173 = Index Array(array=w299, index=4) -> (element=w300:cluster{string[]})
                n174 = call <vilib>:"NT Read String.vi"("Name"=w302) -> ("String"=w301:string)  [unwired: 9 in, 1 out]
                n175 = Unbundle(w300) -> (w296:string[])
                n176 = Match First String(2:w296, 3:w301) -> (0:w297:i32)  [unwired: 1 out]
                n177 = property on="Ring" class="Ring (strict)"("Value"=w297, "Strings []"=w296) -> ()  [unwired: 2 in, 2 out]
                n178 = property on="Ring" class="Ring (strict)"("Visible"=TRUE) -> ()  [unwired: 2 in, 2 out]
                n179 = property on="Slider" class="Slide (strict)"("Visible"=FALSE) -> ()  [unwired: 2 in, 2 out]
              }
              frame Default {
                n180 = property on="Ring" class="Ring (strict)"("Visible"=FALSE) -> ()  [unwired: 2 in, 2 out]
                n181 = property on="Slider" class="Slide (strict)"("Visible"=FALSE) -> ()  [unwired: 2 in, 2 out]
              }
              frame "Brightness  **", "Color Level  **", "Compression  **", "FPS  **", "Sharpness  **" {
                n182 = call <vilib>:"NT Read Number.vi"("Name"=w308) -> ("Numeric"=w307:dbl)  [unwired: 9 in, 1 out]
                n183 = local write "Slider"(w307) -> ()
                n184 = property on="Slider" class="Slide (strict)"("Visible"=TRUE, "Scale.Maximum"=100.0 ("Scale.Range:Maximum")) -> ()  [unwired: 2 in, 2 out]
                n185 = property on="Ring" class="Ring (strict)"("Visible"=FALSE) -> ()  [unwired: 2 in, 2 out]
              }
            }
          }
        }
        n186 = property on="Progress" class="Clust (strict)"("Visible"=FALSE) -> ()  [unwired: 2 in, 2 out]
      }
      event "Test Name": Mouse Enter {
        # "Populate the ring with the list of tests"
        n187 = event-data() -> ()  [unwired: 1 in, 1 out]
        n188 = call <vilib>:"NT Read String Array.vi"("Name"="TestMode/TestList") -> ("String Array"=w315:string[])  [unwired: 9 in, 1 out]
        n189 = Build Array (concatenate)("Select the test to run...", w315) -> (w314:string[])
        n190 = property on="Test Name" class="Ring (strict)"("Strings []"=w314) -> ()  [unwired: 2 in, 2 out]
      }
      event "Test Name": Value Change {
        w317 = FALSE ("Visible")
        # "Tell the robot the test name to run"
        n191 = event-data() -> ("NewVal"=w321:u16)  [unwired: 1 in]
        n192 = property on="Test Name" class="Ring (strict)"() -> ("Strings []"=w322:string[])  [unwired: 2 in, 2 out]
        n193 = local write "Progress"(T4 {"Test Progress"=0, "Test Progress Text"=""} ("Progress")) -> ()
        n194 = Index Array(array=w322, index=w321) -> (element=w320:string)
        n195 = call <vilib>:"NT Write String.vi"("String"=w320, "Name"="TestMode/TestName") -> ()  [unwired: 9 in, 1 out]
        n196 = property on="Progress" class="Clust (strict)"("Visible"=TRUE) -> ()  [unwired: 2 in, 2 out]
        n197 = property on="Motor" class="Clust (strict)"("Visible"=w317) -> ()  [unwired: 2 in, 2 out]
        n198 = property on="Slider" class="Slide (strict)"("Visible"=w317) -> ()  [unwired: 2 in, 2 out]
        n199 = property on="On/Off" class="Bool (strict)"("Visible"=w317) -> ()  [unwired: 2 in, 2 out]
        n200 = property on="Rev/Fwd" class="Clust (strict)"("Visible"=w317) -> ()  [unwired: 2 in, 2 out]
        n201 = property on="Ring" class="Ring (strict)"("Visible"=w317) -> ()  [unwired: 2 in, 2 out]
      }
      event "Listbox": Double Click {
        n202 = event-data() -> ("PlatMods.Shift"=w325:bool, "Row"=w327:i32)  [unwired: 1 in]
        n203 = case shown="False" w325 {
          tunnel: w327 -> [w331 _]
          tunnel: 1 -> [w330 _]
          frame False {
            n204 = property on="Listbox" class="LstBox (strict)"() -> ("Item Symbols"=w329:i32[])  [unwired: 2 in, 2 out]
            n205 = Replace Array Subset(array=w329, new element=w330, index=w331) -> (w328:i32[])
            n206 = property on="Listbox" class="LstBox (strict)"("Item Symbols"=w328) -> ()  [unwired: 2 in, 2 out]
          }
          frame True {
            w332 = 0 ("Top Row")
            n207 = property on="Listbox" class="LstBox (strict)"() -> ("Number of Rows"=w334:u32)  [unwired: 2 in, 2 out]
            n208 = Initialize Array(0, w334) -> (w333:i32[])
            n209 = property on="Listbox" class="LstBox (strict)"("Top Row"=w332, "Value"=w332, "Item Symbols"=w333) -> ()  [unwired: 2 in, 2 out]
          }
        }
      }
      event "Listbox": Key Down {
        n210 = event-data() -> ("VKey"=w338:T18)  [unwired: 1 in]
        n211 = case shown="\"Left\", \"Right\"" w338 {
          selector: w338 -> [w343 _]
          tunnel: eventvkey."Left" ("VKey") -> [w341 _]
          frame "Left", "Right" {
            n212 = Equal?(x=w341, y=w343) -> (x = y?=w342:bool)
            n213 = Select(t=0, s=w342, f=1) -> (s? t:f=w344:i32)
            n214 = property on="Listbox" class="LstBox (strict)"() -> ("Item Symbols"=w347:i32[])  [unwired: 2 in, 2 out]
            n215 = Replace Array Subset(array=w347, new element=w344, index="Listbox") -> (w346:i32[])
            n216 = property on="Listbox" class="LstBox (strict)"("Item Symbols"=w346) -> ()  [unwired: 2 in, 2 out]
          }
          frame Default {
          }
        }
      }
      event "DB Camera Config": Value Change {
        n217 = event-data() -> ("NewVal"=w351:bool)  [unwired: 1 in]
        n218 = case shown="False" w351 {
          tunnel: w350 -> [w360 _]
          tunnel: [w353 w371] -> w349
          tunnel: w348 -> [w352 w371]
          frame False {
            w367 = "Camera"
            w370 = FALSE ("Visible")
            n219 = local read "Camera Settings"() -> (w359:T1)
            n220 = Index Array(array=w360) -> (element=w363:cluster{string[]})  [unwired: 1 in]
            n221 = Unbundle(w359) -> ("Frate Rate"=w358:i32, "Compression"=w357:i32, "Size"=w361:u16)
            n222 = Unbundle(w363) -> (w362:string[])
            n223 = Index Array(array=w362, index=w361) -> (element=w356:string)
            n224 = call-poly <vilib>:"Write Key.vi"("section"=w367, "value"=w356, "key"="Size", "refnum"=w352) -> ("refnum out"=w369:T17)  [unwired: 2 in, 5 out]
            n225 = call-poly <vilib>:"Write Key.vi"("section"=w367, "value"=w358, "key"="FrameRate", "refnum"=w369) -> ("refnum out"=w368:T17)  [unwired: 1 in, 6 out]
            n226 = property on="Camera Settings" class="Clust (strict)"("Visible"=w370) -> ()  [unwired: 2 in, 2 out]
            n227 = local write "DB Camera Config"(w370) -> ()
            n228 = call-poly <vilib>:"Write Key.vi"("section"=w367, "value"=w357, "key"="Compression", "refnum"=w368) -> ("refnum out"=w354:T17)  [unwired: 1 in, 6 out]
            n229 = call <vilib>:"Close Config Data.vi"("refnum"=w354) -> ("file path"=w355:path)  [unwired: 2 in, 8 out]
            n230 = call <vilib>:"Open Config Data.vi"("configuration file path"=w355) -> ("refnum"=w353:T17)  [unwired: 8 in, 2 out]
          }
          frame True {
            n231 = property on="Camera Settings" class="Clust (strict)"("Visible"=TRUE) -> ()  [unwired: 2 in, 2 out]
          }
        }
      }
      event "Camera Settings": Value Change {
        n232 = event-data() -> ("NewVal"=w384:T1)  [unwired: 1 in]
        n233 = Index Array(array=w380) -> (element=w379:cluster{string[]})  [unwired: 1 in]
        n234 = Unbundle(w384) -> ("Frate Rate"=w375:i32, "Compression"=w374:i32, "Size"=w377:u16)
        n235 = Unbundle(w379) -> (w378:string[])
        n236 = Index Array(array=w378, index=w377) -> (element=w376:string)
        n237 = Format Into String(format string="%s   %dfps   %d%%", w376, w375, w374) -> (resulting string=w381:string)  [unwired: 2 in, 1 out]
        n238 = Build Array(w381) -> (w382:string[])
        n239 = property on="DB Camera Config" class="Bool (strict)"("Strings [4]"=w382) -> ()  [unwired: 2 in, 2 out]
      }
      event "Motor.Enable": Value Change {
        n240 = event-data() -> ("NewVal"=w390:bool)  [unwired: 1 in]
        n241 = Unbundle("Motor") -> ("Value"=w389:dbl)  [unwired: 1 out]
        n242 = Select(t=w389, s=w390, f=0.0) -> (s? t:f=w387:dbl)
        n243 = call <vilib>:"NT Write Number.vi"("Numeric"=w387, "Name"=w386) -> ()  [unwired: 9 in, 1 out]
      }
      event "Slider": Value Change {
        n244 = event-data() -> ("NewVal"=w393:dbl)  [unwired: 1 in]
        n245 = call <vilib>:"NT Write Number.vi"("Numeric"=w393, "Name"=w394) -> ()  [unwired: 9 in, 1 out]
      }
      event "On/Off": Value Change {
        n246 = event-data() -> ("NewVal"=w398:bool)  [unwired: 1 in]
        n247 = Boolean To (0,1)(Boolean=w398) -> (0, 1=w397:i16)
        n248 = call <vilib>:"NT Write Number.vi"("Numeric"=w397, "Name"=w396) -> ()  [unwired: 9 in, 1 out]
      }
      event "Rev/Fwd": Value Change {
        n249 = event-data() -> ("NewVal.Forward"=w406:bool, "NewVal.Reverse"=w405:bool)  [unwired: 1 in]
        n250 = Boolean To (0,1)(Boolean=w406) -> (0, 1=w402:i16)
        n251 = Boolean To (0,1)(Boolean=w405) -> (0, 1=w404:i16)
        n252 = Negate(x=w404) -> (-x=w403:i16)
        n253 = Add(x=w402, y=w403) -> (x+y=w401:i16)
        n254 = call <vilib>:"NT Write Number.vi"("Numeric"=w401, "Name"=w400) -> ()  [unwired: 9 in, 1 out]
      }
      event "Ring": Value Change {
        n255 = event-data() -> ("NewVal"=w410:u16)  [unwired: 1 in]
        n256 = property on="Ring" class="Ring (strict)"() -> ("Strings []"=w411:string[])  [unwired: 2 in, 2 out]
        n257 = Index Array(array=w411, index=w410) -> (element=w409:string)
        n258 = call <vilib>:"NT Write String.vi"("String"=w409, "Name"=w408) -> ()  [unwired: 9 in, 1 out]
      }
    }
  }
  n259 = Index Array(array=w13) -> (element=w14:cluster{string[]})  [unwired: 1 in]
  n260 = Unbundle(w14) -> (w12:string[])
  n261 = Match First String(2:w12, 3:w11) -> (0:w10:i32)  [unwired: 1 out]
  n262 = Bundle("value"=w16, "value"=w15, "index"=w10) -> (w4:cluster{"value":i32, "value":i32, "index":i32})  [unwired: 1 out]
  n263 = property on="On/Off" class="Bool (strict)"("Visible"=w27) -> ()  [unwired: 2 in, 2 out]
  n264 = property on="Motor" class="Clust (strict)"("Visible"=w27) -> ()  [unwired: 2 in, 2 out]
  n265 = property on="Progress" class="Clust (strict)"("Visible"=w27) -> ()  [unwired: 2 in, 2 out]
  n266 = property on="Ring" class="Ring (strict)"("Visible"=w27) -> ()  [unwired: 2 in, 2 out]
  n267 = property on="Camera Settings" class="Clust (strict)"("Val(Sgnl)"=w4) -> ()  [unwired: 2 in, 2 out]
  n268 = property on="Rev/Fwd" class="Clust (strict)"("Visible"=w27) -> ()  [unwired: 2 in, 2 out]
  n269 = property on="Camera Settings" class="Clust (strict)"("Visible"=w27) -> ()  [unwired: 2 in, 2 out]
  n270 = local write "DB Camera Config"(w27) -> ()
